vi "Elevator Object Counter.vi"(5 "Clear Stack?":bool, 7 "Toggle Trashcan?":bool, 8 "Trashcan Delta":i32, 10 "Tote Delta":i32) -> (0 "Have Trashcan":bool, 2 "Tote Count":i8)   [LabVIEW 2014]
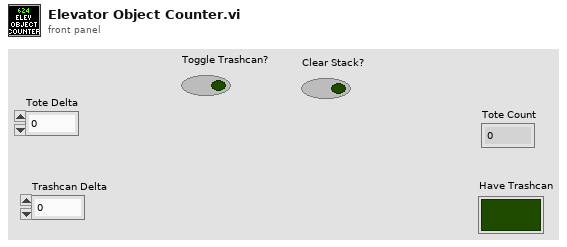
[diagram p1: front panel]
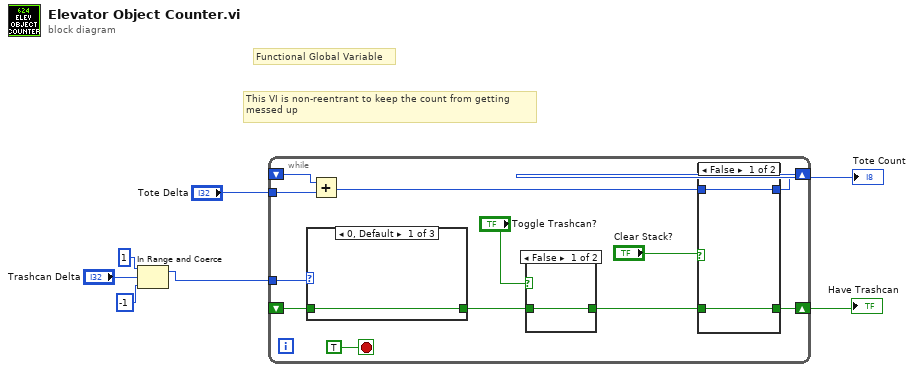
[diagram p0: block diagram]
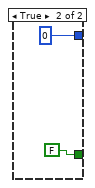
[diagram p2: hidden frame]
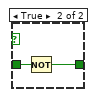
[diagram p3: hidden frame]
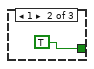
[diagram p4: hidden frame]
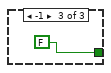
[diagram p5: hidden frame]
diagram:
  # "Functional Global Variable"
  # "This VI is non-reentrant to keep the count from getting\nmessed up"
  n1 = In Range and Coerce(upper limit=1, x="Trashcan Delta", lower limit=-1) -> (coerced(x)=w2:i32)  [unwired: 1 out]
  n2 = while {
    shift-right: [w10] -> w1
    shift-left: _ -> [w15]
    shift-right: [w9] -> w7
    shift-left: _ -> [w18]
    tunnel: "Tote Delta" -> [w17]
    tunnel: w2 -> [w16]
    stop <- TRUE stop-if-true
    n3 = case shown="0, Default" w16 {
      tunnel: [w27 TRUE FALSE] -> w13
      tunnel: w15 -> [w27 _ _]
      frame 0, Default {
      }
      frame 1 {
      }
      frame -1 {
      }
    }
    n4 = Add(x=w18, y=w17) -> (x+y=w8:i32)
    n5 = case shown="False" "Toggle Trashcan?" {
      tunnel: w13 -> [w24 w26]
      tunnel: [w24 w25] -> w11
      frame False {
      }
      frame True {
        n6 = Not(x=w26) -> (.not. x?=w25:bool)
      }
    }
    n7 = case shown="False" "Clear Stack?" {
      tunnel: w11 -> [w20 _]
      tunnel: [w20 FALSE] -> w10
      tunnel: [w21 0] -> w9
      tunnel: w8 -> [w21 _]
      frame False {
      }
      frame True {
      }
    }
  }
  "Have Trashcan" <- w1
  "Tote Count" <- w7
